vi "Draw Frame.vi"(9 "draw options":T1={"Text Color"=16777238, "Wing Color"=16751616, "Dial Outline Color"=13816530, "Sky Color"=3381759, "Ground Color"=8213043, "Horizon Line Color"=16777225, "Outline Color"=0, "Dial Background Color"=5987163, "Draw Wings"=TRUE, "Draw Text"=TRUE, "Font Name"="Helvetica", "Angle units"=enum."Degrees"}, 10 "draw area state":T3, 11 "picture in":picture) -> (3 "picture out":picture)   [LabVIEW 2017, in "NI_Robotics_Attitude Picture.lvlib"]
uses:
  <vilib>/robotics/Controls/Attitude Indicator/Attitude Picture/NI_Robotics_Attitude Picture.lvlib
  <vilib>/robotics/Controls/Attitude Indicator/Attitude Picture/Draw Area State.ctl
  <vilib>/Utility/miscctls.llb/LVBoundsTypeDef.ctl
  <vilib>/robotics/Controls/Attitude Indicator/Attitude Picture/Draw Options.ctl
  <vilib>/robotics/Controls/Utilities/Angle Units.ctl
  <vilib>/robotics/Controls/Utilities/NI_Robotics_Control Utilities.lvlib
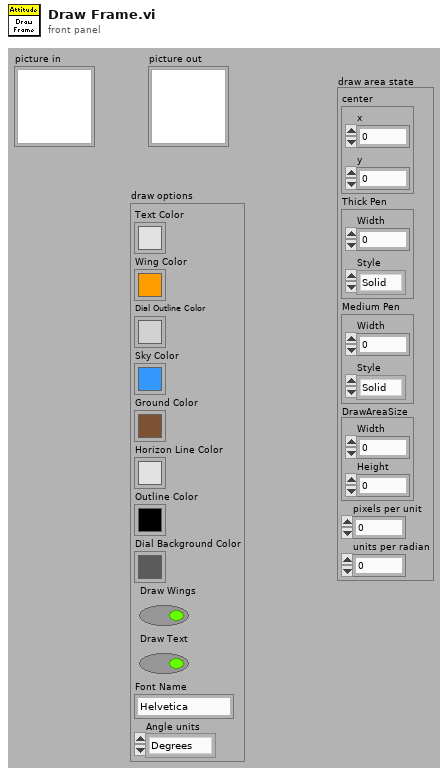
[diagram p1: front panel]
types:
  T1 = typedef "NI_Robotics_Attitude Picture.lvlib/Draw Options.ctl" = cluster{"Text Color":u32, "Wing Color":u32, "Dial Outline Color":u32, "Sky Color":u32, "Ground Color":u32, "Horizon Line Color":u32, "Outline Color":u32, "Dial Background Color":u32, "Draw Wings":bool, "Draw Text":bool, "Font Name":string, "Angle units":T2}
  T2 = typedef "NI_Robotics_Control Utilities.lvlib/Angle Units.ctl" = enum16{"Radians", "Degrees"}
  T3 = typedef "NI_Robotics_Attitude Picture.lvlib/Draw Area State.ctl" = cluster{"center":cluster{"x":i16, "y":i16}, "Thick Pen":cluster{"Width":u16, "Style":enum32{"Solid", "Dash", "Dot", "DashDot", "DashDotDot"}}, "Medium Pen":cluster{"Width":u16, "Style":enum32{"Solid", "Dash", "Dot", "DashDot", "DashDotDot"}}, "DrawAreaSize":T4, "pixels per unit":dbl, "units per radian":dbl}
  T4 = typedef "LVBoundsTypeDef.ctl" = cluster{"Width":u32, "Height":u32}
  T5 = cluster{"Width":u16, "Style":enum32{"Solid", "Dash", "Dot", "DashDot", "DashDotDot"}}
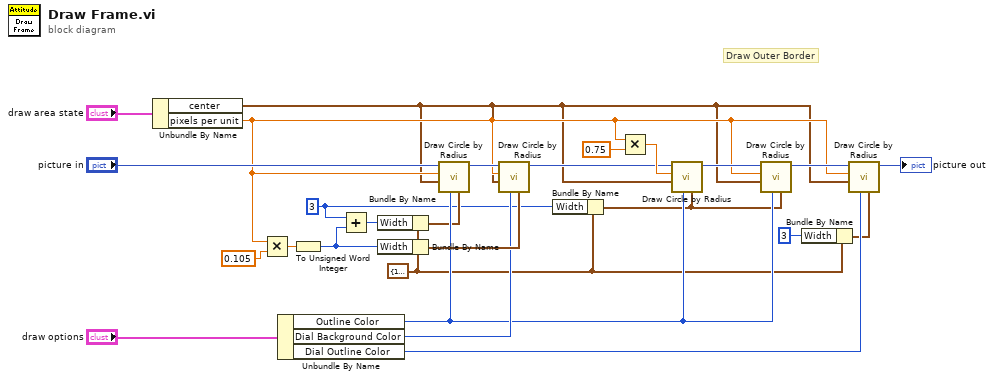
[diagram p0: block diagram]
diagram:
  w5 = u16 3 ("x")
  w2 = T5 {"Width"=1, "Style"=enum."Solid"} ("output cluster")
  # "Draw Outer Border"
  n1 = Unbundle By Name("draw area state") -> ("center"=w11:cluster{"x":i16, "y":i16}, "pixels per unit"=w12:dbl)
  n2 = Multiply(x=w12, y=0.105) -> (x*y=w7:dbl)
  n3 = Unbundle By Name("draw options") -> ("Outline Color"=w10:u32, "Dial Background Color"=w19:u32, "Dial Outline Color"=w18:u32)
  n4 = To Unsigned Word Integer(number=w7) -> (unsigned 16bit integer=w4:u16)
  n5 = Add(x=w5, y=w4) -> (x+y=w8:u16)
  n6 = Bundle By Name(cluster=w2, "Width"=w8) -> (w9:T5)
  n7 = Bundle By Name(cluster=w2, "Width"=w4) -> (w23:T5)
  n8 = call <vilib>:"Draw Circle by Radius.vi"("pen"=w9, "color(black)"=w10, "pixel center"=w11, "radius"=w12, "picture"="picture in") -> ("new picture"=w13:picture)  [unwired: 6 in]
  n9 = call <vilib>:"Draw Circle by Radius.vi"("pen"=w23, "color(black)"=w19, "pixel center"=w11, "radius"=w12, "picture"=w13) -> ("new picture"=w16:picture)  [unwired: 6 in]
  n10 = Bundle By Name(cluster=w2, "Width"=w5) -> (w6:T5)
  n11 = Multiply(x=w12, y=0.75 ("Frame Width")) -> (x*y=w22:dbl)
  n12 = call <vilib>:"Draw Circle by Radius.vi"("pen"=w6, "color(black)"=w10, "pixel center"=w11, "radius"=w22, "picture"=w16) -> ("new picture"=w15:picture)  [unwired: 6 in]
  n13 = call <vilib>:"Draw Circle by Radius.vi"("pen"=w6, "color(black)"=w10, "pixel center"=w11, "radius"=w12, "picture"=w15) -> ("new picture"=w25:picture)  [unwired: 6 in]
  n14 = Bundle By Name(cluster=w2, "Width"=u16 3) -> (w3:T5)
  n15 = call <vilib>:"Draw Circle by Radius.vi"("pen"=w3, "color(black)"=w18, "pixel center"=w11, "radius"=w12, "picture"=w25) -> ("new picture"=→"picture out":picture)  [unwired: 6 in]
